vi "simpletls test platsock.vi"() -> ()   [LabVIEW 2016]
uses:
  libretls/context parent/lvlibretls configurable context.lvclass/lvlibretls configurable context.ctl
  libretls/client/lvlibretls client socket.lvclass
  C:/Users/IEUser/Desktop/tlssimple/libretls/context parent/lvlibretls configurable context.lvclass
  libretls/context parent/lvlibretls configurable context.lvclass
  libretls/lv tls dll.lvlib
panel:
  out "return":i32
  out "error out":errorcluster
  out "data":string
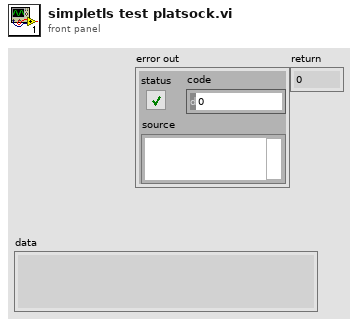
[diagram p1: front panel]
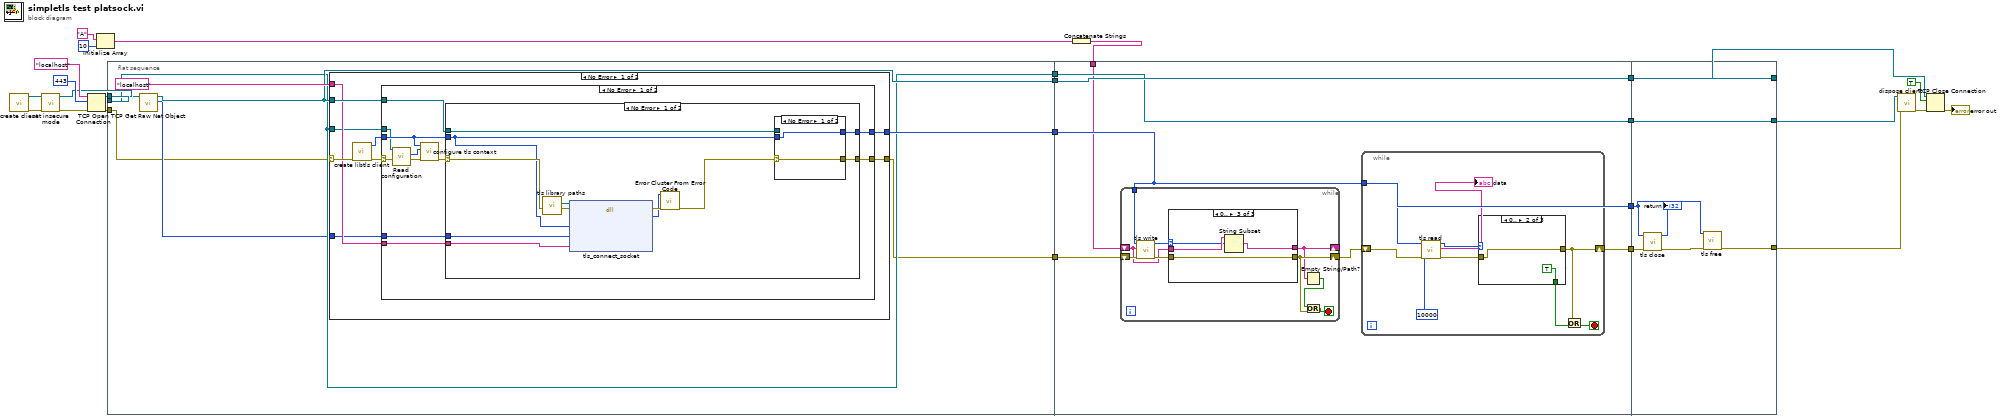
[diagram p0: block diagram]
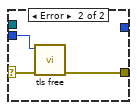
[diagram p2: hidden frame]
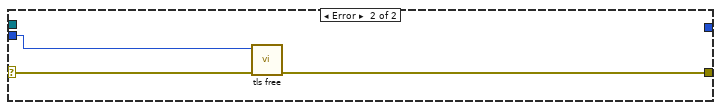
[diagram p3: hidden frame]
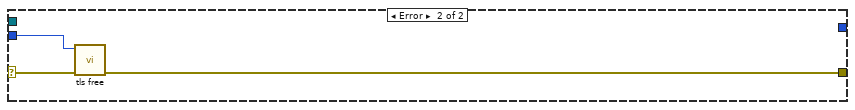
[diagram p4: hidden frame]
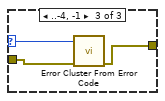
[diagram p7: hidden frame]
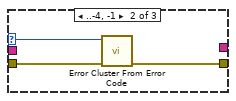
[diagram p9: hidden frame]
diagram:
  n1 = call "create client.vi"() -> ("error out"=w18:errorcluster, "lvlibretls client socket out"=w14:refnum<class "lvlibretls client socket.lvclass">)  [unwired: 10 in]
  n2 = call "set insecure mode.vi"("error in"=w18, "lvlibretls configurable context in"=w14) -> ("error out"=w15:errorcluster, "lvlibretls configurable context out"=w13:refnum<class "lvlibretls client socket.lvclass">)  [unwired: 8 in]
  n3 = TCP Open Connection(address="localhost", remote port or service name=u16 443, error in (no error)=w15) -> (connection ID=w16:refnum<k5>, error out=w17:errorcluster)  [unwired: 2 in]
  n4 = Initialize Array("A" ("address"), 10 ("dimension size")) -> (w22:string[])
  n5 = flat-sequence {
    tunnel: w17 -> [w27]
    tunnel: w16 -> [w34]
    tunnel: w13 -> [w30]
    tunnel: [w32] -> w11
    tunnel: [w30] -> w10
    tunnel: [w31] -> w5
    tunnel: [w29] -> w1
    tunnel: w11 -> [w83]
    tunnel: w10 -> [w82]
    tunnel: [w83] -> w8
    tunnel: [w82] -> w7
    tunnel: [w81] -> w6
    tunnel: w5 -> [w79]
    tunnel: [w79] -> w4
    tunnel: w2 -> [w78]
    tunnel: w1 -> [w77]
    tunnel: [w122] -> w9
    tunnel: [w123] -> w12
    tunnel: w8 -> [w123]
    tunnel: w7 -> [w122]
    tunnel: w6 -> [w120]
    tunnel: w4 -> [w119]
    tunnel: [w118] -> w3
    frame #0 {
      n6 = call <vilib>:"TCP Get Raw Net Object.vi"("connection ID"=w34) -> ("raw net object"=w28:u64, "connection ID out"=w32:refnum<k5>)  [unwired: 8 in, 1 out]
      n7 = case shown="No Error" w27 {
        selector: w27 -> [w40 w76]
        tunnel: [w43 w76] -> w29
        tunnel: w32 -> [w42 _]
        tunnel: "localhost" ("server name") -> [w38 _]
        tunnel: w28 -> [w37 _]
        tunnel: [w36 _] -> w31
        tunnel: w30 -> [w35 _]
        frame No Error {
          n8 = call "create libtls client.vi"("error in"=w40) -> ("error out"=w41:errorcluster, "client out"=w39:u64)  [unwired: 9 in]
          n9 = case shown="No Error" w41 {
            selector: w41 -> [w51 w75]
            tunnel: [w53 w74] -> w43
            tunnel: w42 -> [w52 _]
            tunnel: w39 -> [w49 w73]
            tunnel: w38 -> [w48 _]
            tunnel: w37 -> [w47 _]
            tunnel: [w46 _] -> w36
            tunnel: w35 -> [w44 _]
            frame No Error {
              n10 = call "Read configuration.vi"("lvlibretls configurable context in"=w44) -> ("configuration"=w45:u64)  [unwired: 10 in]
              n11 = call "configure tls context.vi"("error in"=w51, "config"=w45, "context"=w49) -> ("error out"=w50:errorcluster)  [unwired: 8 in]
              n12 = case shown="No Error" w50 {
                selector: w50 -> [w60 w72]
                tunnel: [w63 w71] -> w53
                tunnel: w52 -> [w64 _]
                tunnel: w49 -> [w58 w70]
                tunnel: w48 -> [w57 _]
                tunnel: w47 -> [w55 _]
                tunnel: [w54 _] -> w46
                frame No Error {
                  n13 = call "tls library paths.vi"() -> ("libtls"=w56:path)  [unwired: 8 in, 3 out]
                  n14 = dll-call lib="C:/Users/IEUser/Desktop/tlssimple/libtls-15.dll" fn="tls_connect_socket"(path in=w56, error in=w60, "context"=w58, "socket"=w55, "servername"=w57) -> (error out=w62:errorcluster, "err"=w61:i32)  [unwired: 4 in, 1 out]
                  n15 = call <vilib>:"Error Cluster From Error Code.vi"("error in (no error)"=w62, "error code (0)"=w61) -> ("error out"=w59:errorcluster)  [unwired: 7 in]
                  n16 = case shown="No Error" w59 {
                    selector: w59 -> [w66 w69]
                    tunnel: w64 -> [_ _]
                    tunnel: w58 -> [w65 w68]
                    tunnel: [w66 w67] -> w63
                    tunnel: [w65 _] -> w54
                    frame No Error {
                    }
                    frame Error {
                      n17 = call "tls free.vi"("error in"=w69, "tls context"=w68) -> ("error out"=w67:errorcluster)  [unwired: 9 in]
                    }
                  }
                }
                frame Error {
                  n18 = call "tls free.vi"("error in"=w72, "tls context"=w70) -> ("error out"=w71:errorcluster)  [unwired: 9 in]
                }
              }
            }
            frame Error {
              n19 = call "tls free.vi"("error in"=w75, "tls context"=w73) -> ("error out"=w74:errorcluster)  [unwired: 9 in]
            }
          }
        }
        frame Error {
        }
      }
    }
    frame #1 {
      n20 = while {
        tunnel: w79 -> [w107]
        shift-right: [w102] -> w80
        shift-left: w77 -> [w106]
        shift-right: [w100] -> _
        shift-left: w78 -> [w103]
        stop <- w101 stop-if-true
        n21 = call "tls write.vi"("error in"=w106, "data"=w103, "tls context"=w107) -> ("error out"=w104:errorcluster, "error response"=w105:i32)  [unwired: 7 in]
        n22 = case shown="0.." w105 {
          selector: w105 -> [_ w110 w113]
          tunnel: [w108 w111 w116] -> w102
          tunnel: w104 -> [w108 w112 w116]
          tunnel: w103 -> [w109 _ w115]
          tunnel: [w109 _ w114] -> w100
          frame -3, -2 {
          }
          frame ..-4, -1 {
            n23 = call <vilib>:"Error Cluster From Error Code.vi"("error in (no error)"=w112, "error code (0)"=w110) -> ("error out"=w111:errorcluster)  [unwired: 7 in]
          }
          frame 0.. {
            n24 = String Subset(string=w115, offset (0)=w113) -> (substring=w114:string)  [unwired: 1 in]
          }
        }
        n25 = Empty String/Path?(string/path=w100) -> (empty?=w99:bool)
        n26 = Or(x=w99, y=w102) -> (x .or. y?=w101:bool)
      }
      n27 = while {
        tunnel: w79 -> [w91]
        shift-right: [w84] -> w81
        shift-left: w80 -> [w92]
        stop <- w86 stop-if-true
        n28 = call "tls read.vi"("error in"=w92, "max read size"=u64 10000, "tls context"=w91) -> ("error out"=w85:errorcluster, "buffer"=→"data":string, "error response"=w88:i32)  [unwired: 6 in]
        n29 = case shown="0.." w88 {
          selector: w88 -> [_ _ w96]
          tunnel: [_ TRUE _] -> w87
          tunnel: w85 -> [w93 w94 w98]
          tunnel: [w93 w94 w97] -> w84
          frame -3, -2 {
          }
          frame 0.. {
          }
          frame ..-4, -1 {
            n30 = call <vilib>:"Error Cluster From Error Code.vi"("error in (no error)"=w98, "error code (0)"=w96) -> ("error out"=w97:errorcluster)  [unwired: 7 in]
          }
        }
        n31 = Or(x=w84, y=w87) -> (x .or. y?=w86:bool)
      }
    }
    frame #2 {
      n32 = call "tls close.vi"("error in"=w120, "tls context"=w119) -> ("error out"=w121:errorcluster, "return"=→"return":i32)  [unwired: 8 in]
      n33 = call "tls free.vi"("error in"=w121, "tls context"=w119) -> ("error out"=w118:errorcluster)  [unwired: 9 in]
    }
  }
  n34 = Concatenate Strings(w22) -> (w2:string)
  n35 = call "dispose client.vi"("error in"=w3, "lvlibretls client socket in"=w9) -> ("error out"=w19:errorcluster)  [unwired: 9 in]
  n36 = TCP Close Connection(connection ID=w12, abort (F)=TRUE, error in (no error)=w19) -> (error out=→"error out":errorcluster)  [unwired: 1 out]
